vi "dataUserIn.vi"(8 "error in (no error)":errorcluster, 10 "password":string, 11 "username":string) -> (0 "error out":errorcluster)   [LabVIEW 2014]
panel:
  out "连接的字符串":string
  in  "is_administrator":u16(ring) items=["True", "False"]
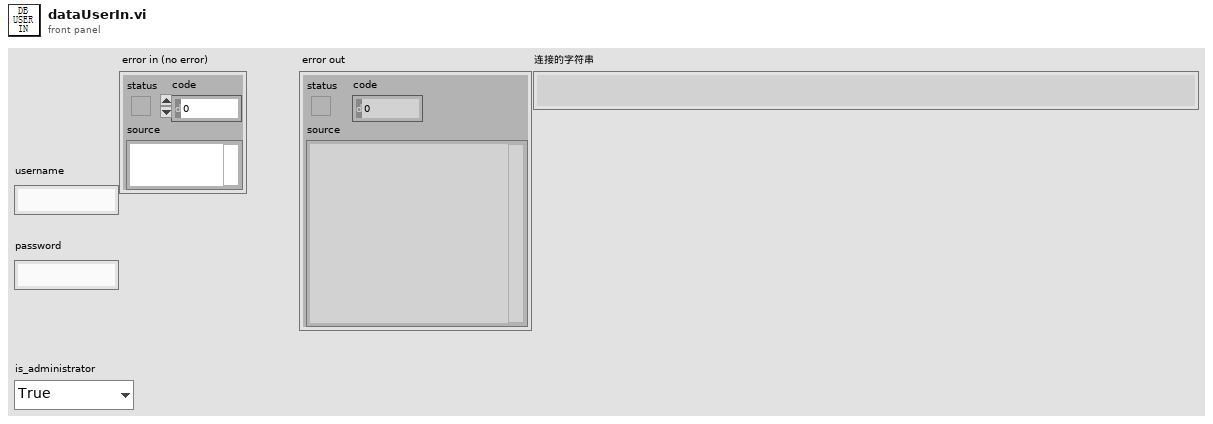
[diagram p1: front panel]
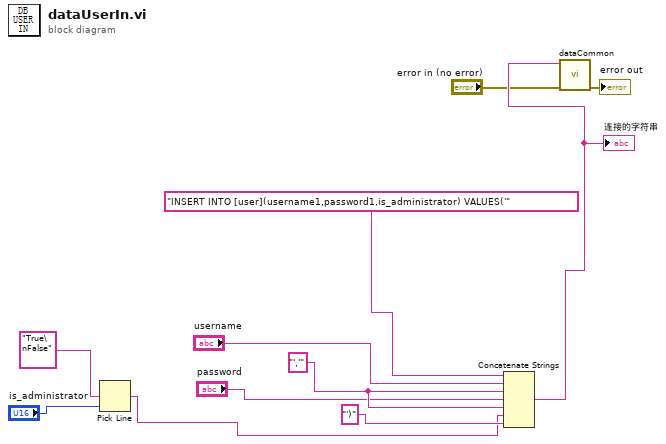
[diagram p0: block diagram]
diagram:
  w10 = "','"
  n1 = Pick Line(multi-line string="True\nFalse" ("多行字符串"), line index="is_administrator") -> (output string=w1:string)  [unwired: 1 in]
  n2 = Concatenate Strings("INSERT INTO [user](username1,password1,is_administrator) VALUES('", "username", w10, "password", w10, w1, "')") -> (w6:string)
  "连接的字符串" <- w6
  n3 = call "dataCommon.vi"("error in (no error)"="error in (no error)", "Command Text"=w6) -> ("error out"=→"error out":errorcluster)  [unwired: 8 in, 1 out]
